vi "Is Local.vi"(8 "error in (no error)":errorcluster, 11 "Guardian in":refnum<class "Guardian.lvclass">) -> (0 "error out":errorcluster, 2 "Is Local?":bool, 3 "Guardian out":refnum<class "Guardian.lvclass">)   [LabVIEW 2026]
uses:
  Guardian.lvclass
  C:/LabVIEW Code/TALOS/talos/Ancestor/Ancestor/Ancestor.lvclass
  Ancestor/Ancestor/Ancestor.lvclass/Ancestor.ctl
  Ancestor/Ancestor/Read ID.vi
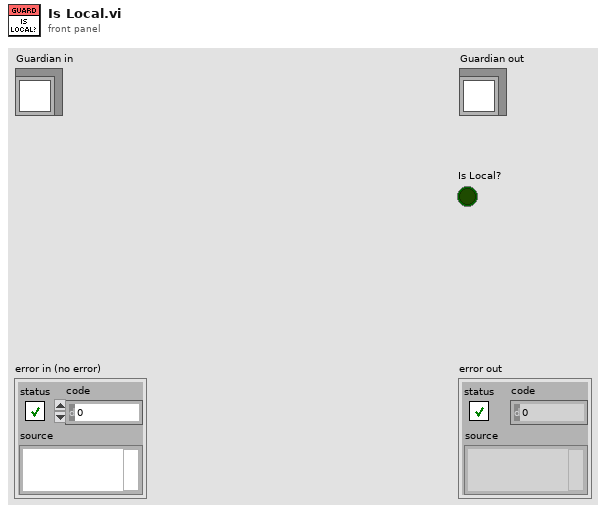
[diagram p1: front panel]
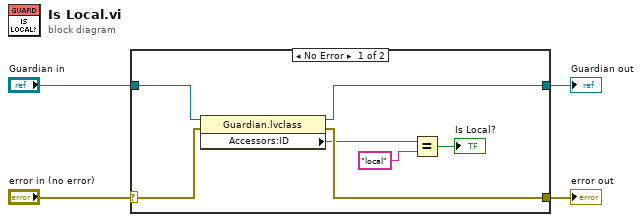
[diagram p0: block diagram]
diagram:
  n1 = case shown="No Error" "error in (no error)" {
    selector: "error in (no error)" -> [w9 w13]
    tunnel: [w8 w13] -> w3
    tunnel: [w11 w12] -> w1
    tunnel: "Guardian in" -> [w10 w12]
    frame No Error {
      n2 = property class="Guardian.lvclass"(reference=w10, error in=w9) -> (reference out=w11:refnum<class "Guardian.lvclass">, error out=w8:errorcluster, "Accessors:ID"=w6:string)
      n3 = Equal?(x=w6, y="local") -> (x = y?=→"Is Local?":bool)
    }
    frame Error {
    }
  }
  "error out" <- w3
  "Guardian out" <- w1
